vi "Get Status Pin6.vi"(8 "error in (no error)":errorcluster, 11 "index":i32) -> (0 "error out":errorcluster, 2 "status out":i32, 3 "index_out":i32)   [LabVIEW 2010, in "FEMTO_LUCI-10.lvlib"]
doc: "This function reads status of PIN 6."
uses:
  <userlib>/FEMTO/FEMTO_LUCI-10.lvlib
  <userlib>/FEMTO/LUCI_10.dll
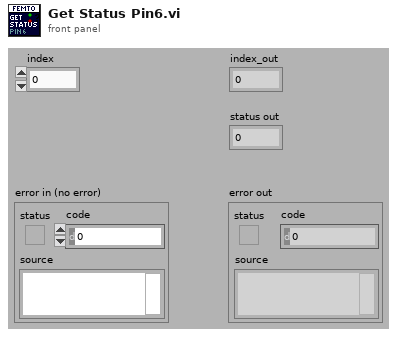
[diagram p1: front panel]
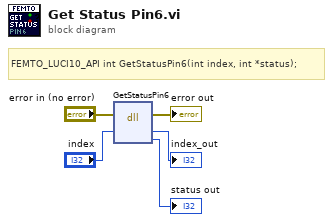
[diagram p0: block diagram]
diagram:
  # "FEMTO_LUCI10_API int GetStatusPin6(int index, int *status);"
  n1 = dll-call lib="C:/Program Files (x86)/National Instruments/LabVIEW 2010/user.lib/FEMTO/LUCI_10.*" fn="GetStatusPin6"(error in="error in (no error)", "index"="index") -> (error out=→"error out":errorcluster, "index"=→"index_out":i32, "status"=→"status out":i32)  [unwired: 2 in, 3 out]
